vi "toI32.vi"(8 "error in (no error)":errorcluster, 11 "Value":variant) -> (0 "error out":errorcluster, 3 "id":i32)   [LabVIEW 2018, in "Account History.lvclass"]
uses:
  Account History.lvclass
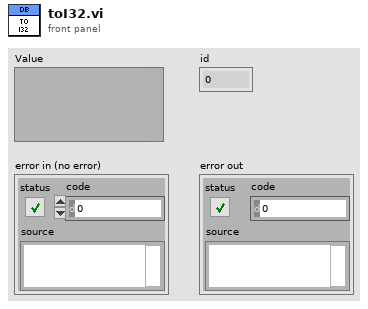
[diagram p1: front panel]
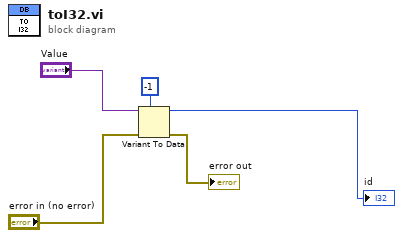
[diagram p0: block diagram]
diagram:
  n1 = Variant To Data(error in="error in (no error)", type=-1 ("id"), Variant="Value") -> (data=→"id":i32, error out=→"error out":errorcluster)
